vi "canDataSort.vi"() -> ()   [LabVIEW 2023] (continued)
00000004    8        68\t00\t97\tCC\t00\t16\t39\t78\r\n      1882  1FFFFFFF   00000004    8        00\t20\tFF\tFF\tFF\tFF\tFF\tFF\r\n      1872  1FFFFFFF   00000004    8        00\t20\tFF\tFF\tFF\tFF\tFF\tFF\r\n      1863  0CF102A7   00000004    8        30\t75\tE0\t2E\t80\tFF\tFF\tFD\r\n      1863  0CF101A7   00000004    8        68\t00\t97\tCC\t00\t16\t39\t77\r\n      1862  1FFFFFFF   00000004    8        00\t20\tFF\tFF\tFF\tFF\tFF\tFF\r\n      1852  1FFFFFFF   00000004    8        00\t20\tFF\tFF\tFF\tFF\tFF\tFF\r\n      1847  1FFFFFFF   00000004    8        00\t00\tFF\tFF\tFF\tFF\tFF\tFF\r\n      1846  18F121F0   00000004    8        09\t18\t00\t00\tFF\tFF\tB0\t01\r\n      1845  18F106A7   00000004    8        00\tF7\tFF\tFF\tFF\tFF\tFF\t95\r\n      1892  1FFFFFFF   00000004    8        00\t00\tFF\tFF\tFF\tFF\tFF\tFF\r\n      1883  0CF102A7   00000004    8        30\t75\tE0\t2E\t80\tFF\tFF\tFD\r\n      1883  0CF101A7   00000004    8        68\t00\t97\tCC\t00\t16\t39\t78\r\n      1882  1FFFFFFF   00000004    8        00\t20\tFF\tFF\tFF\tFF\tFF\tFF\r\n      1872  1FFFFFFF   00000004    8        00\t20\tFF\tFF\tFF\tFF\tFF\tFF\r\n      1863  0CF102A7   00000004    8        30\t75\tE0\t2E\t80\tFF\tFF\tFD\r\n      1863  0CF101A7   00000004    8        68\t00\t97\tCC\t00\t16\t39\t77\r\n      1862  1FFFFFFF   00000004    8        00\t20\tFF\tFF\tFF\tFF\tFF\tFF\r\n      1852  1FFFFFFF   00000004    8        00\t20\tFF\tFF\tFF\tFF\tFF\tFF\r\n      1847  1FFFFFFF   00000004    8        00\t00\tFF\tFF\tFF\tFF\tFF\tFF\r\n      1846  18F121F0   00000004    8        09\t18\t00\t00\tFF\tFF\tB0\t01\r\n      1893  18F106A7   00000004    8        00\tF7\tFF\tFF\tFF\tFF\tFF\t96\r\n      1892  1FFFFFFF   00000004    8        00\t00\tFF\tFF\tFF\tFF\tFF\tFF\r\n      1883  0CF102A7   00000004    8        30\t75\tE0\t2E\t80\tFF\tFF\tFD\r\n      1883  0CF101A7   00000004    8        68\t00\t97\tCC\t00\t16\t39\t78\r\n      1882  1FFFFFFF   00000004    8        00\t20\tFF\tFF\tFF\tFF\tFF\tFF\r\n      1872  1FFFFFFF   00000004    8        00\t20\tFF\tFF\tFF\tFF\tFF\tFF\r\n      1863  0CF102A7   00000004    8        30\t75\tE0\t2E\t80\tFF\tFF\tFD\r\n      1863  0CF101A7   00000004    8        68\t00\t97\tCC\t00\t16\t39\t77\r\n      1862  1FFFFFFF   00000004    8        00\t20\tFF\tFF\tFF\tFF\tFF\tFF\r\n      1852  1FFFFFFF   00000004    8        00\t20\tFF\tFF\tFF\tFF\tFF\tFF\r\n      1847  1FFFFFFF   00000004    8        00\t00\tFF\tFF\tFF\tFF\tFF\tFF\r\n      1902  1FFFFFFF   00000004    8        00\t20\tFF\tFF\tFF\tFF\tFF\tFF\r\n      1893  18F106A7   00000004    8        00\tF7\tFF\tFF\tFF\tFF\tFF\t96\r\n      1892  1FFFFFFF   00000004    8        00\t00\tFF\tFF\tFF\tFF\tFF\tFF\r\n      1883  0CF102A7   00000004    8        30\t75\tE0\t2E\t80\tFF\tFF\tFD\r\n      1883  0CF101A7   00000004    8        68\t00\t97\tCC\t00\t16\t39\t78\r\n      1882  1FFFFFFF   00000004    8        00\t20\tFF\tFF\tFF\tFF\tFF\tFF\r\n      1872  1FFFFFFF   00000004    8        00\t20\tFF\tFF\tFF\tFF\tFF\tFF\r\n      1863  0CF102A7   00000004    8        30\t75\tE0\t2E\t80\tFF\tFF\tFD\r\n      1863  0CF101A7   00000004    8        68\t00\t97\tCC\t00\t16\t39\t77\r\n      1862  1FFFFFFF   00000004    8        00\t20\tFF\tFF\tFF\tFF\tFF\tFF\r\n      1852  1FFFFFFF   00000004    8        00\t20\tFF\tFF\tFF\tFF\tFF\tFF\r\n      1903  0CF101A7   00000004    8        68\t00\t97\tCC\t00\t16\t39\t79\r\n      1902  1FFFFFFF   00000004    8        00\t20\tFF\tFF\tFF\tFF\tFF\tFF\r\n      1893  18F106A7   00000004    8        00\tF7\tFF\tFF\tFF\tFF\tFF\t96\r\n      1892  1FFFFFFF   00000004    8        00\t00\tFF\tFF\tFF\tFF\tFF\tFF\r\n      1883  0CF102A7   00000004    8        30\t75\tE0\t2E\t80\tFF\tFF\tFD\r\n      1883  0CF101A7   00000004    8        68\t00\t97\tCC\t00\t16\t39\t78\r\n      1882  1FFFFFFF   00000004    8        00\t20\tFF\tFF\tFF\tFF\tFF\tFF\r\n      1872  1FFFFFFF   00000004    8        00\t20\tFF\tFF\tFF\tFF\tFF\tFF\r\n      1863  0CF102A7   00000004    8        30\t75\tE0\t2E\t80\tFF\tFF\tFD\r\n      1863  0CF101A7   00000004    8        68\t00\t97\tCC\t00\t16\t39\t77\r\n      1862  1FFFFFFF   00000004    8        00\t20\tFF\tFF\tFF\tFF\tFF\tFF\r\n      1903  0CF102A7   00000004    8        30\t75\tE0\t2E\t80\tFF\tFF\tFD\r\n      1903  0CF101A7   00000004    8        68\t00\t97\tCC\t00\t16\t39\t79\r\n      1902  1FFFFFFF   00000004    8        00\t20\tFF\tFF\tFF\tFF\tFF\tFF\r\n      1893  18F106A7   00000004    8        00\tF7\tFF\tFF\tFF\tFF\tFF\t96\r\n      1892  1FFFFFFF   00000004    8        00\t00\tFF\tFF\tFF\tFF\tFF\tFF\r\n      1883  0CF102A7   00000004    8        30\t75\tE0\t2E\t80\tFF\tFF\tFD\r\n      1883  0CF101A7   00000004    8        68\t00\t97\tCC\t00\t16\t39\t78\r\n      1882  1FFFFFFF   00000004    8        00\t20\tFF\tFF\tFF\tFF\tFF\tFF\r\n      1872  1FFFFFFF   00000004    8        00\t20\tFF\tFF\tFF\tFF\tFF\tFF\r\n      1863  0CF102A7   00000004    8        30\t75\tE0\t2E\t80\tFF\tFF\tFD\r\n      1863  0CF101A7   00000004    8        68\t00\t97\tCC\t00\t16\t39\t77\r\n      1912  1FFFFFFF   00000004    8        00\t00\tFF\tFF\tFF\tFF\tFF\tFF\r\n      1903  0CF102A7   00000004    8        30\t75\tE0\t2E\t80\tFF\tFF\tFD\r\n      1903  0CF101A7   00000004    8        68\t00\t97\tCC\t00\t16\t39\t79\r\n      1902  1FFFFFFF   00000004    8        00\t20\tFF\tFF\tFF\tFF\tFF\tFF\r\n      1893  18F106A7   00000004    8        00\tF7\tFF\tFF\tFF\tFF\tFF\t96\r\n      1892  1FFFFFFF   00000004    8        00\t00\tFF\tFF\tFF\tFF\tFF\tFF\r\n      1883  0CF102A7   00000004    8        30\t75\tE0\t2E\t80\tFF\tFF\tFD\r\n      1883  0CF101A7   00000004    8        68\t00\t97\tCC\t00\t16\t39\t78\r\n      1882  1FFFFFFF   00000004    8        00\t20\tFF\tFF\tFF\tFF\tFF\tFF\r\n      1872  1FFFFFFF   00000004    8        00\t20\tFF\tFF\tFF\tFF\tFF\tFF\r\n      1863  0CF102A7   00000004    8        30\t75\tE0\t2E\t80\tFF\tFF\tFD\r\n      1922  1FFFFFFF   00000004    8        00\t20\tFF\tFF\tFF\tFF\tFF\tFF\r\n      1912  1FFFFFFF   00000004    8        00\t00\tFF\tFF\tFF\tFF\tFF\tFF\r\n      1903  0CF102A7   00000004    8        30\t75\tE0\t2E\t80\tFF\tFF\tFD\r\n      1903  0CF101A7   00000004    8        68\t00\t97\tCC\t00\t16\t39\t79\r\n      1902  1FFFFFFF   00000004    8        00\t20\tFF\tFF\tFF\tFF\tFF\tFF\r\n      1893  18F106A7   00000004    8        00\tF7\tFF\tFF\tFF\tFF\tFF\t96\r\n      1892  1FFFFFFF   00000004    8        00\t00\tFF\tFF\tFF\tFF\tFF\tFF\r\n      1883  0CF102A7   00000004    8        30\t75\tE0\t2E\t80\tFF\tFF\tFD\r\n      1883  0CF101A7   00000004    8        68\t00\t97\tCC\t00\t16\t39\t78\r\n      1882  1FFFFFFF   00000004    8        00\t20\tFF\tFF\tFF\tFF\tFF\tFF\r\n      1872  1FFFFFFF   00000004    8        00\t20\tFF\tFF\tFF\tFF\tFF\tFF\r\n      1923  0CF101A7   00000004    8        68\t00\t97\tCC\t00\t16\t39\t7A\r\n      1922  1FFFFFFF   00000004    8        00\t20\tFF\tFF\tFF\tFF\tFF\tFF\r\n      1912  1FFFFFFF   00000004    8        00\t00\tFF\tFF\tFF\tFF\tFF\tFF\r\n      1903  0CF102A7   00000004    8        30\t75\tE0\t2E\t80\tFF\tFF\tFD\r\n      1903  0CF101A7   00000004    8        68\t00\t97\tCC\t00\t16\t39\t79\r\n      1902  1FFFFFFF   00000004    8        00\t20\tFF\tFF\tFF\tFF\tFF\tFF\r\n      1893  18F106A7   00000004    8        00\tF7\tFF\tFF\tFF\tFF\tFF\t96\r\n      1892  1FFFFFFF   00000004    8        00\t00\tFF\tFF\tFF\tFF\tFF\tFF\r\n      1883  0CF102A7   00000004    8        30\t75\tE0\t2E\t80\tFF\tFF\tFD\r\n      1883  0CF101A7   00000004    8        68\t00\t97\tCC\t00\t16\t39\t78\r\n      1882  1FFFFFFF   00000004    8        00\t20\tFF\tFF\tFF\tFF\tFF\tFF\r\n      1923  0CF102A7   00000004    8        30\t75\tE0\t2E\t80\tFF\tFF\tFD\r\n      1923  0CF101A7   00000004    8        68\t00\t97\tCC\t00\t16\t39\t7A\r\n      1922  1FFFFFFF   00000004    8        00\t20\tFF\tFF\tFF\tFF\tFF\tFF\r\n      1912  1FFFFFFF   00000004    8        00\t00\tFF\tFF\tFF\tFF\tFF\tFF\r\n      1903  0CF102A7   00000004    8        30\t75\tE0\t2E\t80\tFF\tFF\tFD\r\n      1903  0CF101A7   00000004    8        68\t00\t97\tCC\t00\t16\t39\t79\r\n      1902  1FFFFFFF   00000004    8        00\t20\tFF\tFF\tFF\tFF\tFF\tFF\r\n      1893  18F106A7   00000004    8        00\tF7\tFF\tFF\tFF\tFF\tFF\t96\r\n      1892  1FFFFFFF   00000004    8        00\t00\tFF\tFF\tFF\tFF\tFF\tFF\r\n      1883  0CF102A7   00000004    8        30\t75\tE0\t2E\t80\tFF\tFF\tFD\r\n      1883  0CF101A7   00000004    8        68\t00\t97\tCC\t00\t16\t39\t78\r\n      1932  1FFFFFFF   00000004    8        00\t20\tFF\tFF\tFF\tFF\tFF\tFF\r\n      1923  0CF102A7   00000004    8        30\t75\tE0\t2E\t80\tFF\tFF\tFD\r\n      1923  0CF101A7   00000004    8        68\t00\t97\tCC\t00\t16\t39\t7A\r\n      1922  1FFFFFFF   00000004    8        00\t20\tFF\tFF\tFF\tFF\tFF\tFF\r\n      1912  1FFFFFFF   00000004    8        00\t00\tFF\tFF\tFF\tFF\tFF\tFF\r\n      1903  0CF102A7   00000004    8        30\t75\tE0\t2E\t80\tFF\tFF\tFD\r\n      1903  0CF101A7   00000004    8        68\t00\t97\tCC\t00\t16\t39\t79\r\n      1902  1FFFFFFF   00000004    8        00\t20\tFF\tFF\tFF\tFF\tFF\tFF\r\n      1893  18F106A7   00000004    8        00\tF7\tFF\tFF\tFF\tFF\tFF\t96\r\n      1892  1FFFFFFF   00000004    8        00\t00\tFF\tFF\tFF\tFF\tFF\tFF\r\n      1883  0CF102A7   00000004    8        30\t75\tE0\t2E\t80\tFF\tFF\tFD\r\n      1941  18F11FF0   00000004    8        FF\t3F\t90\t68\t88\t1B\t10\tBC\r\n      1932  1FFFFFFF   00000004    8        00\t20\tFF\tFF\tFF\tFF\tFF\tFF\r\n      1923  0CF102A7   00000004    8        30\t75\tE0\t2E\t80\tFF\tFF\tFD\r\n      1923  0CF101A7   00000004    8        68\t00\t97\tCC\t00\t16\t39\t7A\r\n      1922  1FFFFFFF   00000004    8        00\t20\tFF\tFF\tFF\tFF\tFF\tFF\r\n      1912  1FFFFFFF   00000004    8        00\t00\tFF\tFF\tFF\tFF\tFF\tFF\r\n      1903  0CF102A7   00000004    8        30\t75\tE0\t2E\t80\tFF\tFF\tFD\r\n      1903  0CF101A7   00000004    8        68\t00\t97\tCC\t00\t16\t39\t79\r\n      1902  1FFFFFFF   00000004    8        00\t20\tFF\tFF\tFF\tFF\tFF\tFF\r\n      1893  18F106A7   00000004    8        00\tF7\tFF\tFF\tFF\tFF\tFF\t96\r\n      1892  1FFFFFFF   00000004    8        00\t00\tFF\tFF\tFF\tFF\tFF\tFF\r\n      1942  18F120F0   00000004    8        2B\t75\t60\tB1\tB0\t01\tFF\tFF\r\n      1941  18F11FF0   00000004    8        FF\t3F\t90\t68\t88\t1B\t10\tBC\r\n      1932  1FFFFFFF   00000004    8        00\t20\tFF\tFF\tFF\tFF\tFF\tFF\r\n      1923  0CF102A7   00000004    8        30\t75\tE0\t2E\t80\tFF\tFF\tFD\r\n      1923  0CF101A7   00000004    8        68\t00\t97\tCC\t00\t16\t39\t7A\r\n      1922  1FFFFFFF   00000004    8        00\t20\tFF\tFF\tFF\tFF\tFF\tFF\r\n      1912  1FFFFFFF   00000004    8        00\t00\tFF\tFF\tFF\tFF\tFF\tFF\r\n      1903  0CF102A7   00000004    8        30\t75\tE0\t2E\t80\tFF\tFF\tFD\r\n      1903  0CF101A7   00000004    8        68\t00\t97\tCC\t00\t16\t39\t79\r\n      1902  1FFFFFFF   00000004    8        00\t20\tFF\tFF\tFF\tFF\tFF\tFF\r\n      1893  18F106A7   00000004    8        00\tF7\tFF\tFF\tFF\tFF\tFF\t96\r\n      1943  0CF101A7   00000004    8        68\t00\t97\tCC\t00\t16\t39\t7B\r\n      1942  18F120F0   00000004    8        2B\t75\t60\tB1\tB0\t01\tFF\tFF\r\n      1941  18F11FF0   00000004    8        FF\t3F\t90\t68\t88\t1B\t10\tBC\r\n      1932  1FFFFFFF   00000004    8        00\t20\tFF\tFF\tFF\tFF\tFF\tFF\r\n      1923  0CF102A7   00000004    8        30\t75\tE0\t2E\t80\tFF\tFF\tFD\r\n      1923  0CF101A7   00000004    8        68\t00\t97\tCC\t00\t16\t39\t7A\r\n      1922  1FFFFFFF   00000004    8        00\t20\tFF\tFF\tFF\tFF\tFF\tFF\r\n      1912  1FFFFFFF   00000004    8        00\t00\tFF\tFF\tFF\tFF\tFF\tFF\r\n      1903  0CF102A7   00000004    8        30\t75\tE0\t2E\t80\tFF\tFF\tFD\r\n      1903  0CF101A7   00000004    8        68\t00\t97\tCC\t00\t16\t39\t79\r\n      1902  1FFFFFFF   00000004    8        00\t20\tFF\tFF\tFF\tFF\tFF\tFF\r\n      1943  0C3C4D4A   00000004    8        BE\tFF\tFF\t7F\t18\tFF\tFF\t4B\r\n      1943  0CF101A7   00000004    8        68\t00\t97\tCC\t00\t16\t39\t7B\r\n      1942  18F120F0   00000004    8        2B\t75\t60\tB1\tB0\t01\tFF\tFF\r\n      1941  18F11FF0   00000004    8        FF\t3F\t90\t68\t88\t1B\t10\tBC\r\n      1932  1FFFFFFF   00000004    8        00\t20\tFF\tFF\tFF\tFF\tFF\tFF\r\n      1923  0CF102A7   00000004    8        30\t75\tE0\t2E\t80\tFF\tFF\tFD\r\n      1923  0CF101A7   00000004    8        68\t00\t97\tCC\t00\t16\t39\t7A\r\n      1922  1FFFFFFF   00000004    8        00\t20\tFF\tFF\tFF\tFF\tFF\tFF\r\n      1912  1FFFFFFF   00000004    8        00\t00\tFF\tFF\tFF\tFF\tFF\tFF\r\n      1903  0CF102A7   00000004    8        30\t75\tE0\t2E\t80\tFF\tFF\tFD\r\n      1903  0CF101A7   00000004    8        68\t00\t97\tCC\t00\t16\t39\t79\r\n      1944  0CF102A7   00000004    8        30\t75\tE0\t2E\t80\tFF\tFF\tFD\r\n      1943  0C3C4D4A   00000004    8        BE\tFF\tFF\t7F\t18\tFF\tFF\t4B\r\n      1943  0CF101A7   00000004    8        68\t00\t97\tCC\t00\t16\t39\t7B\r\n      1942  18F120F0   00000004    8        2B\t75\t60\tB1\tB0\t01\tFF\tFF\r\n      1941  18F11FF0   00000004    8        FF\t3F\t90\t68\t88\t1B\t10\tBC\r\n      1932  1FFFFFFF   00000004    8        00\t20\tFF\tFF\tFF\tFF\tFF\tFF\r\n      1923  0CF102A7   00000004    8        30\t75\tE0\t2E\t80\tFF\tFF\tFD\r\n      1923  0CF101A7   00000004    8        68\t00\t97\tCC\t00\t16\t39\t7A\r\n      1922  1FFFFFFF   00000004    8        00\t20\tFF\tFF\tFF\tFF\tFF\tFF\r\n      1912  1FFFFFFF   00000004    8        00\t00\tFF\tFF\tFF\tFF\tFF\tFF\r\n      1903  0CF102A7   00000004    8        30\t75\tE0\t2E\t80\tFF\tFF\tFD\r\n      1944  0CF103A7   00000004    8        17\t1F\t08\t60\tB1\t1F\t08\t4B\r\n      1944  0CF102A7   00000004    8        30\t75\tE0\t2E\t80\tFF\tFF\tFD\r\n      1943  0C3C4D4A   00000004    8        BE\tFF\tFF\t7F\t18\tFF\tFF\t4B\r\n      1943  0CF101A7   00000004    8        68\t00\t97\tCC\t00\t16\t39\t7B\r\n      1942  18F120F0   00000004    8        2B\t75\t60\tB1\tB0\t01\tFF\tFF\r\n      1941  18F11FF0   00000004    8        FF\t3F\t90\t68\t88\t1B\t10\tBC\r\n      1932  1FFFFFFF   00000004    8        00\t20\tFF\tFF\tFF\tFF\tFF\tFF\r\n      1923  0CF102A7   00000004    8        30\t75\tE0\t2E\t80\tFF\tFF\tFD\r\n      1923  0CF101A7   00000004    8        68\t00\t97\tCC\t00\t16\t39\t7A\r\n      1922  1FFFFFFF   00000004    8        00\t20\tFF\tFF\tFF\tFF\tFF\tFF\r\n      1912  1FFFFFFF   00000004    8        00\t00\tFF\tFF\tFF\tFF\tFF\tFF\r\n      1945  0CF104A7   00000004    8        F0\t60\t22\tFC\tFF\tFF\tFF\t4B\r\n      1944  0CF103A7   00000004    8        17\t1F\t08\t60\tB1\t1F\t08\t4B\r\n      1944  0CF102A7   00000004    8        30\t75\tE0\t2E\t80\tFF\tFF\tFD\r\n      1943  0C3C4D4A   00000004    8        BE\tFF\tFF\t7F\t18\tFF\tFF\t4B\r\n      1943  0CF101A7   00000004    8        68\t00\t97\tCC\t00\t16\t39\t7B\r\n      1942  18F120F0   00000004    8        2B\t75\t60\tB1\tB0\t01\tFF\tFF\r\n      1941  18F11FF0   00000004    8        FF\t3F\t90\t68\t88\t1B\t10\tBC\r\n      1932  1FFFFFFF   00000004    8        00\t20\tFF\tFF\tFF\tFF\tFF\tFF\r\n      1923  0CF102A7   00000004    8        30\t75\tE0\t2E\t80\tFF\tFF\tFD\r\n      1923  0CF101A7   00000004    8        68\t00\t97\tCC\t00\t16\t39\t7A\r\n      1922  1FFFFFFF   00000004    8        00\t20\tFF\tFF\tFF\tFF\tFF\tFF\r\n      1945  18F106A7   00000004    8        00\tF7\tFF\tFF\tFF\tFF\tFF\t97\r\n      1945  0CF104A7   00000004    8        F0\t60\t22\tFC\tFF\tFF\tFF\t4B\r\n      1944  0CF103A7   00000004    8        17\t1F\t08\t60\tB1\t1F\t08\t4B\r\n      1944  0CF102A7   00000004    8        30\t75\tE0\t2E\t80\tFF\tFF\tFD\r\n      1943  0C3C4D4A   00000004    8        BE\tFF\tFF\t7F\t18\tFF\tFF\t4B\r\n      1943  0CF101A7   00000004    8        68\t00\t97\tCC\t00\t16\t39\t7B\r\n      1942  18F120F0   00000004    8        2B\t75\t60\tB1\tB0\t01\tFF\tFF\r\n      1941  18F11FF0   00000004    8        FF\t3F\t90\t68\t88\t1B\t10\tBC\r\n      1932  1FFFFFFF   00000004    8        00\t20\tFF\tFF\tFF\tFF\tFF\tFF\r\n      1923  0CF102A7   00000004    8        30\t75\tE0\t2E\t80\tFF\tFF\tFD\r\n      1923  0CF101A7   00000004    8        68\t00\t97\tCC\t00\t16\t39\t7A\r\n      1946  18F121F0   00000004    8        09\t18\t00\t00\tFF\tFF\tB0\t01\r\n      1945  18F106A7   00000004    8        00\tF7\tFF\tFF\tFF\tFF\tFF\t97\r\n      1945  0CF104A7   00000004    8        F0\t60\t22\tFC\tFF\tFF\tFF\t4B\r\n      1944  0CF103A7   00000004    8        17\t1F\t08\t60\tB1\t1F\t08\t4B\r\n      1944  0CF102A7   00000004    8        30\t75\tE0\t2E\t80\tFF\tFF\tFD\r\n      1943  0C3C4D4A   00000004    8        BE\tFF\tFF\t7F\t18\tFF\tFF\t4B\r\n      1943  0CF101A7   00000004    8        68\t00\t97\tCC\t00\t16\t39\t7B\r\n      1942  18F120F0   00000004    8        2B\t75\t60\tB1\tB0\t01\tFF\tFF\r\n      1941  18F11FF0   00000004    8        FF\t3F\t90\t68\t88\t1B\t10\tBC\r\n      1932  1FFFFFFF   00000004    8        00\t20\tFF\tFF\tFF\tFF\tFF\tFF\r\n      1923  0CF102A7   00000004    8        30\t75\tE0\t2E\t80\tFF\tFF\tFD\r\n      1947  1FFFFFFF   00000004    8        00\t20\tFF\tFF\tFF\tFF\tFF\tFF\r\n      1946  18F121F0   00000004    8        09\t18\t00\t00\tFF\tFF\tB0\t01\r\n      1945  18F106A7   00000004    8        00\tF7\tFF\tFF\tFF\tFF\tFF\t97\r\n      1945  0CF104A7   00000004    8        F0\t60\t22\tFC\tFF\tFF\tFF\t4B\r\n      1944  0CF103A7   00000004    8        17\t1F\t08\t60\tB1\t1F\t08\t4B\r\n      1944  0CF102A7   00000004    8        30\t75\tE0\t2E\t80\tFF\tFF\tFD\r\n      1943  0C3C4D4A   00000004    8        BE\tFF\tFF\t7F\t18\tFF\tFF\t4B\r\n      1943  0CF101A7   00000004    8        68\t00\t97\tCC\t00\t16\t39\t7B\r\n      1942  18F120F0   00000004    8        2B\t75\t60\tB1\tB0\t01\tFF\tFF\r\n      1941  18F11FF0   00000004    8        FF\t3F\t90\t68\t88\t1B\t10\tBC\r\n      1932  1FFFFFFF   00000004    8        00\t20\tFF\tFF\tFF\tFF\tFF\tFF\r\n      1952  1FFFFFFF   00000004    8        00\t00\tFF\tFF\tFF\tFF\tFF\tFF\r\n      1947  1FFFFFFF   00000004    8        00\t20\tFF\tFF\tFF\tFF\tFF\tFF\r\n      1946  18F121F0   00000004    8        09\t18\t00\t00\tFF\tFF\tB0\t01\r\n      1945  18F106A7   00000004    8        00\tF7\tFF\tFF\tFF\tFF\tFF\t97\r\n      1945  0CF104A7   00000004    8        F0\t60\t22\tFC\tFF\tFF\tFF\t4B\r\n      1944  0CF103A7   00000004    8        17\t1F\t08\t60\tB1\t1F\t08\t4B\r\n      1944  0CF102A7   00000004    8        30\t75\tE0\t2E\t80\tFF\tFF\tFD\r\n      1943  0C3C4D4A   00000004    8        BE\tFF\tFF\t7F\t18\tFF\tFF\t4B\r\n      1943  0CF101A7   00000004    8        68\t00\t97\tCC\t00\t16\t39\t7B\r\n      1942  18F120F0   00000004    8        2B\t75\t60\tB1\tB0\t01\tFF\tFF\r\n      1941  18F11FF0   00000004    8        FF\t3F\t90\t68\t88\t1B\t10\tBC\r\n      1962  1FFFFFFF   00000004    8        00\t00\tFF\tFF\tFF\tFF\tFF\tFF\r\n      1952  1FFFFFFF   00000004    8        00\t00\tFF\tFF\tFF\tFF\tFF\tFF\r\n      1947  1FFFFFFF   00000004    8        00\t20\tFF\tFF\tFF\tFF\tFF\tFF\r\n      1946  18F121F0   00000004    8        09\t18\t00\t00\tFF\tFF\tB0\t01\r\n      1945  18F106A7   00000004    8        00\tF7\tFF\tFF\tFF\tFF\tFF\t97\r\n      1945  0CF104A7   00000004    8        F0\t60\t22\tFC\tFF\tFF\tFF\t4B\r\n      1944  0CF103A7   00000004    8        17\t1F\t08\t60\tB1\t1F\t08\t4B\r\n      1944  0CF102A7   00000004    8        30\t75\tE0\t2E\t80\tFF\tFF\tFD\r\n      1943  0C3C4D4A   00000004    8        BE\tFF\tFF\t7F\t18\tFF\tFF\t4B\r\n      1943  0CF101A7   00000004    8        68\t00\t97\tCC\t00\t16\t39\t7B\r\n      1942  18F120F0   00000004    8        2B\t75\t60\tB1\tB0\t01\tFF\tFF\r\n      1963  0CF101A7   00000004    8        68\t00\t97\tCC\t00\t16\t39\t7C\r\n      1962  1FFFFFFF   00000004    8        00\t00\tFF\tFF\tFF\tFF\tFF\tFF\r\n      1952  1FFFFFFF   00000004    8        00\t00\tFF\tFF\tFF\tFF\tFF\tFF\r\n      1947  1FFFFFFF   00000004    8        00\t20\tFF\tFF\tFF\tFF\tFF\tFF\r\n      1946  18F121F0   00000004    8        09\t18\t00\t00\tFF\tFF\tB0\t01\r\n      1945  18F106A7   00000004    8        00\tF7\tFF\tFF\tFF\tFF\tFF\t97\r\n      1945  0CF104A7   00000004    8        F0\t60\t22\tFC\tFF\tFF\tFF\t4B\r\n      1944  0CF103A7   00000004    8        17\t1F\t08\t60\tB1\t1F\t08\t4B\r\n      1944  0CF102A7   00000004    8        30\t75\tE0\t2E\t80\tFF\tFF\tFD\r\n      1943  0C3C4D4A   00000004    8        BE\tFF\tFF\t7F\t18\tFF\tFF\t4B\r\n      1943  0CF101A7   00000004    8        68\t00\t97\tCC\t00\t16\t39\t7B\r\n      1963  0CF102A7   00000004    8        30\t75\tE0\t2E\t80\tFF\tFF\tFD\r\n      1963  0CF101A7   00000004    8        68\t00\t97\tCC\t00\t16\t39\t7C\r\n      1962  1FFFFFFF   00000004    8        00\t00\tFF\tFF\tFF\tFF\tFF\tFF\r\n      1952  1FFFFFFF   00000004    8        00\t00\tFF\tFF\tFF\tFF\tFF\tFF\r\n      1947  1FFFFFFF   00000004    8        00\t20\tFF\tFF\tFF\tFF\tFF\tFF\r\n      1946  18F121F0   00000004    8        09\t18\t00\t00\tFF\tFF\tB0\t01\r\n      1945  18F106A7   00000004    8        00\tF7\tFF\tFF\tFF\tFF\tFF\t97\r\n      1945  0CF104A7   00000004    8        F0\t60\t22\tFC\tFF\tFF\tFF\t4B\r\n      1944  0CF103A7   00000004    8        17\t1F\t08\t60\tB1\t1F\t08\t4B\r\n      1944  0CF102A7   00000004    8        30\t75\tE0\t2E\t80\tFF\tFF\tFD\r\n      1943  0C3C4D4A   00000004    8        BE\tFF\tFF\t7F\t18\tFF\tFF\t4B\r\n      1972  1FFFFFFF   00000004    8        00\t00\tFF\tFF\tFF\tFF\tFF\tFF\r\n      1963  0CF102A7   00000004    8        30\t75\tE0\t2E\t80\tFF\tFF\tFD\r\n      1963  0CF101A7   00000004    8        68\t00\t97\tCC\t00\t16\t39\t7C\r\n      1962  1FFFFFFF   00000004    8        00\t00\tFF\tFF\tFF\tFF\tFF\tFF\r\n      1952  1FFFFFFF   00000004    8        00\t00\tFF\tFF\tFF\tFF\tFF\tFF\r\n      1947  1FFFFFFF   00000004    8        00\t20\tFF\tFF\tFF\tFF\tFF\tFF\r\n      1946  18F121F0   00000004    8        09\t18\t00\t00\tFF\tFF\tB0\t01\r\n      1945  18F106A7   00000004    8        00\tF7\tFF\tFF\tFF\tFF\tFF\t97\r\n      1945  0CF104A7   00000004    8        F0\t60\t22\tFC\tFF\tFF\tFF\t4B\r\n      1944  0CF103A7   00000004    8        17\t1F\t08\t60\tB1\t1F\t08\t4B\r\n      1944  0CF102A7   00000004    8        30\t75\tE0\t2E\t80\tFF\tFF\tFD\r\n      1982  1FFFFFFF   00000004    8        00\t20\tFF\tFF\tFF\tFF\tFF\tFF\r\n      1972  1FFFFFFF   00000004    8        00\t00\tFF\tFF\tFF\tFF\tFF\tFF\r\n      1963  0CF102A7   00000004    8        30\t75\tE0\t2E\t80\tFF\tFF\tFD\r\n      1963  0CF101A7   00000004    8        68\t00\t97\tCC\t00\t16\t39\t7C\r\n      1962  1FFFFFFF   00000004    8        00\t00\tFF\tFF\tFF\tFF\tFF\tFF\r\n      1952  1FFFFFFF   00000004    8        00\t00\tFF\tFF\tFF\tFF\tFF\tFF\r\n      1947  1FFFFFFF   00000004    8        00\t20\tFF\tFF\tFF\tFF\tFF\tFF\r\n      1946  18F121F0   00000004    8        09\t18\t00\t00\tFF\tFF\tB0\t01\r\n      1945  18F106A7   00000004    8        00\tF7\tFF\tFF\tFF\tFF\tFF\t97\r\n      1945  0CF104A7   00000004    8        F0\t60\t22\tFC\tFF\tFF\tFF\t4B\r\n      1944  0CF103A7   00000004    8        17\t1F\t08\t60\tB1\t1F\t08\t4B\r\n      1983  0CF101A7   00000004    8        68\t00\t97\tCC\t00\t16\t39\t7D\r\n      1982  1FFFFFFF   00000004    8        00\t20\tFF\tFF\tFF\tFF\tFF\tFF\r\n      1972  1FFFFFFF   00000004    8        00\t00\tFF\tFF\tFF\tFF\tFF\tFF\r\n      1963  0CF102A7   00000004    8        30\t75\tE0\t2E\t80\tFF\tFF\tFD\r\n      1963  0CF101A7   00000004    8        68\t00\t97\tCC\t00\t16\t39\t7C\r\n      1962  1FFFFFFF   00000004    8        00\t00\tFF\tFF\tFF\tFF\tFF\tFF\r\n      1952  1FFFFFFF   00000004    8        00\t00\tFF\tFF\tFF\tFF\tFF\tFF\r\n      1947  1FFFFFFF   00000004    8        00\t20\tFF\tFF\tFF\tFF\tFF\tFF\r\n      1946  18F121F0   00000004    8        09\t18\t00\t00\tFF\tFF\tB0\t01\r\n      1945  18F106A7   00000004    8        00\tF7\tFF\tFF\tFF\tFF\tFF\t97\r\n      1945  0CF104A7   00000004    8        F0\t60\t22\tFC\tFF\tFF\tFF\t4B\r\n      1983  0CF102A7   00000004    8        30\t75\tE0\t2E\t80\tFF\tFF\tFD\r\n      1983  0CF101A7   00000004    8        68\t00\t97\tCC\t00\t16\t39\t7D\r\n      1982  1FFFFFFF   00000004    8        00\t20\tFF\tFF\tFF\tFF\tFF\tFF\r\n      1972  1FFFFFFF   00000004    8        00\t00\tFF\tFF\tFF\tFF\tFF\tFF\r\n      1963  0CF102A7   00000004    8        30\t75\tE0\t2E\t80\tFF\tFF\tFD\r\n      1963  0CF101A7   00000004    8        68\t00\t97\tCC\t00\t16\t39\t7C\r\n      1962  1FFFFFFF   00000004    8        00\t00\tFF\tFF\tFF\tFF\tFF\tFF\r\n      1952  1FFFFFFF   00000004    8        00\t00\tFF\tFF\tFF\tFF\tFF\tFF\r\n      1947  1FFFFFFF   00000004    8        00\t20\tFF\tFF\tFF\tFF\tFF\tFF\r\n      1946  18F121F0   00000004    8        09\t18\t00\t00\tFF\tFF\tB0\t01\r\n      1945  18F106A7   00000004    8        00\tF7\tFF\tFF\tFF\tFF\tFF\t97\r\n      1992  1FFFFFFF   00000004    8        00\t00\tFF\tFF\tFF\tFF\tFF\tFF\r\n      1983  0CF102A7   00000004    8        30\t75\tE0\t2E\t80\tFF\tFF\tFD\r\n      1983  0CF101A7   00000004    8        68\t00\t97\tCC\t00\t16\t39\t7D\r\n      1982  1FFFFFFF   00000004    8        00\t20\tFF\tFF\tFF\tFF\tFF\tFF\r\n      1972  1FFFFFFF   00000004    8        00\t00\tFF\tFF\tFF\tFF\tFF\tFF\r\n      1963  0CF102A7   00000004    8        30\t75\tE0\t2E\t80\tFF\tFF\tFD\r\n      1963  0CF101A7   00000004    8        68\t00\t97\tCC\t00\t16\t39\t7C\r\n      1962  1FFFFFFF   00000004    8        00\t00\tFF\tFF\tFF\tFF\tFF\tFF\r\n      1952  1FFFFFFF   00000004    8        00\t00\tFF\tFF\tFF\tFF\tFF\tFF\r\n      1947  1FFFFFFF   00000004    8        00\t20\tFF\tFF\tFF\tFF\tFF\tFF\r\n      1946  18F121F0   00000004    8        09\t18\t00\t00\tFF\tFF\tB0\t01\r\n      1993  18F106A7   00000004    8        00\tF7\tFF\tFF\tFF\tFF\tFF\t98\r\n      1992  1FFFFFFF   00000004    8        00\t00\tFF\tFF\tFF\tFF\tFF\tFF\r\n      1983  0CF102A7   00000004    8        30\t75\tE0\t2E\t80\tFF\tFF\tFD\r\n      1983  0CF101A7   00000004    8        68\t00\t97\tCC\t00\t16\t39\t7D\r\n      1982  1FFFFFFF   00000004    8        00\t20\tFF\tFF\tFF\tFF\tFF\tFF\r\n      1972  1FFFFFFF   00000004    8        00\t00\tFF\tFF\tFF\tFF\tFF\tFF\r\n      1963  0CF102A7   00000004    8        30\t75\tE0\t2E\t80\tFF\tFF\tFD\r\n      1963  0CF101A7   00000004    8        68\t00\t97\tCC\t00\t16\t39\t7C\r\n      1962  1FFFFFFF   00000004    8        00\t00\tFF\tFF\tFF\tFF\tFF\tFF\r\n      1952  1FFFFFFF   00000004    8        00\t00\tFF\tFF\tFF\tFF\tFF\tFF\r\n      1947  1FFFFFFF   00000004    8        00\t20\tFF\tFF\tFF\tFF\tFF\tFF\r\n      2002  1FFFFFFF   00000004    8        00\t00\tFF\tFF\tFF\tFF\tFF\tFF\r\n      1993  18F106A7   00000004    8        00\tF7\tFF\tFF\tFF\tFF\tFF\t98\r\n      1992  1FFFFFFF   00000004    8        00\t00\tFF\tFF\tFF\tFF\tFF\tFF\r\n      1983  0CF102A7   00000004    8        30\t75\tE0\t2E\t80\tFF\tFF\tFD\r\n      1983  0CF101A7   00000004    8        68\t00\t97\tCC\t00\t16\t39\t7D\r\n      1982  1FFFFFFF   00000004    8        00\t20\tFF\tFF\tFF\tFF\tFF\tFF\r\n      1972  1FFFFFFF   00000004    8        00\t00\tFF\tFF\tFF\tFF\tFF\tFF\r\n      1963  0CF102A7   00000004    8        30\t75\tE0\t2E\t80\tFF\tFF\tFD\r\n      1963  0CF101A7   00000004    8        68\t00\t97\tCC\t00\t16\t39\t7C\r\n      1962  1FFFFFFF   00000004    8        00\t00\tFF\tFF\tFF\tFF\tFF\tFF\r\n      1952  1FFFFFFF   00000004    8        00\t00\tFF\tFF\tFF\tFF\tFF\tFF\r\n      2003  0CF101A7   00000004    8        68\t00\t97\tCC\t00\t16\t39\t7E\r\n      2002  1FFFFFFF   00000004    8        00\t00\tFF\tFF\tFF\tFF\tFF\tFF\r\n      1993  18F106A7   00000004    8        00\tF7\tFF\tFF\tFF\tFF\tFF\t98\r\n      1992  1FFFFFFF   00000004    8        00\t00\tFF\tFF\tFF\tFF\tFF\tFF\r\n      1983  0CF102A7   00000004    8        30\t75\tE0\t2E\t80\tFF\tFF\tFD\r\n      1983  0CF101A7   00000004    8        68\t00\t97\tCC\t00\t16\t39\t7D\r\n      1982  1FFFFFFF   00000004    8        00\t20\tFF\tFF\tFF\tFF\tFF\tFF\r\n      1972  1FFFFFFF   00000004    8        00\t00\tFF\tFF\tFF\tFF\tFF\tFF\r\n      1963  0CF102A7   00000004    8        30\t75\tE0\t2E\t80\tFF\tFF\tFD\r\n      1963  0CF101A7   00000004    8        68\t00\t97\tCC\t00\t16\t39\t7C\r\n      1962  1FFFFFFF   00000004    8        00\t00\tFF\tFF\tFF\tFF\tFF\tFF\r\n      2003  0CF102A7   00000004    8        30\t75\tE0\t2E\t80\tFF\tFF\tFD\r\n      2003  0CF101A7   00000004    8        68\t00\t97\tCC\t00\t16\t39\t7E\r\n      2002  1FFFFFFF   00000004    8        00\t00\tFF\tFF\tFF\tFF\tFF\tFF\r\n      1993  18F106A7   00000004    8        00\tF7\tFF\tFF\tFF\tFF\tFF\t98\r\n      1992  1FFFFFFF   00000004    8        00\t00\tFF\tFF\tFF\tFF\tFF\tFF\r\n      1983  0CF102A7   00000004    8        30\t75\tE0\t2E\t80\tFF\tFF\tFD\r\n      1983  0CF101A7   00000004    8        68\t00\t97\tCC\t00\t16\t39\t7D\r\n      1982  1FFFFFFF   00000004    8        00\t20\tFF\tFF\tFF\tFF\tFF\tFF\r\n      1972  1FFFFFFF   00000004    8        00\t00\tFF\tFF\tFF\tFF\tFF\tFF\r\n      1963  0CF102A7   00000004    8        30\t75\tE0\t2E\t80\tFF\tFF\tFD\r\n      1963  0CF101A7   00000004    8        68\t00\t97\tCC\t00\t16\t39\t7C\r\n      2012  1FFFFFFF   00000004    8        00\t00\tFF\tFF\tFF\tFF\tFF\tFF\r\n      2003  0CF102A7   00000004    8        30\t75\tE0\t2E\t80\tFF\tFF\tFD\r\n      2003  0CF101A7   00000004    8        68\t00\t97\tCC\t00\t16\t39\t7E\r\n      2002  1FFFFFFF   00000004    8        00\t00\tFF\tFF\tFF\tFF\tFF\tFF\r\n      1993  18F106A7   00000004    8        00\tF7\tFF\tFF\tFF\tFF\tFF\t98\r\n      1992  1FFFFFFF   00000004    8        00\t00\tFF\tFF\tFF\tFF\tFF\tFF\r\n      1983  0CF102A7   00000004    8        30\t75\tE0\t2E\t80\tFF\tFF\tFD\r\n      1983  0CF101A7   00000004    8        68\t00\t97\tCC\t00\t16\t39\t7D\r\n      1982  1FFFFFFF   00000004    8        00\t20\tFF\tFF\tFF\tFF\tFF\tFF\r\n      1972  1FFFFFFF   00000004    8        00\t00\tFF\tFF\tFF\tFF\tFF\tFF\r\n      1963  0CF102A7   00000004    8        30\t75\tE0\t2E\t80\tFF\tFF\tFD\r\n      2022  1FFFFFFF   00000004    8        00\t00\tFF\tFF\tFF\tFF\tFF\tFF\r\n      2012  1FFFFFFF   00000004    8        00\t00\tFF\tFF\tFF\tFF\tFF\tFF\r\n      2003  0CF102A7   00000004    8        30\t75\tE0\t2E\t80\tFF\tFF\tFD\r\n      2003  0CF101A7   00000004    8        68\t00\t97\tCC\t00\t16\t39\t7E\r\n      2002  1FFFFFFF   00000004    8        00\t00\tFF\tFF\tFF\tFF\tFF\tFF\r\n      1993  18F106A7   00000004    8        00\tF7\tFF\tFF\tFF\tFF\tFF\t98\r\n      1992  1FFFFFFF   00000004    8        00\t00\tFF\tFF\tFF\tFF\tFF\tFF\r\n      1983  0CF102A7   00000004    8        30\t75\tE0\t2E\t80\tFF\tFF\tFD\r\n      1983  0CF101A7   00000004    8        68\t00\t97\tCC\t00\t16\t39\t7D\r\n      1982  1FFFFFFF   00000004    8        00\t20\tFF\tFF\tFF\tFF\tFF\tFF\r\n      1972  1FFFFFFF   00000004    8        00\t00\tFF\tFF\tFF\tFF\tFF\tFF\r\n      2023  0CF101A7   00000004    8        68\t00\t97\tCC\t00\t16\t39\t7F\r\n      2022  1FFFFFFF   00000004    8        00\t00\tFF\tFF\tFF\tFF\tFF\tFF\r\n      2012  1FFFFFFF   00000004    8        00\t00\tFF\tFF\tFF\tFF\tFF\tFF\r\n      2003  0CF102A7   00000004    8        30\t75\tE0\t2E\t80\tFF\tFF\tFD\r\n      2003  0CF101A7   00000004    8        68\t00\t97\tCC\t00\t16\t39\t7E\r\n      2002  1FFFFFFF   00000004    8        00\t00\tFF\tFF\tFF\tFF\tFF\tFF\r\n      1993  18F106A7   00000004    8        00\tF7\tFF\tFF\tFF\tFF\tFF\t98\r\n      1992  1FFFFFFF   00000004    8        00\t00\tFF\tFF\tFF\tFF\tFF\tFF\r\n      1983  0CF102A7   00000004    8        30\t75\tE0\t2E\t80\tFF\tFF\tFD\r\n      1983  0CF101A7   00000004    8        68\t00\t97\tCC\t00\t16\t39\t7D\r\n      1982  1FFFFFFF   00000004    8        00\t20\tFF\tFF\tFF\tFF\tFF\tFF\r\n      2023  0CF102A7   00000004    8        30\t75\tE0\t2E\t80\tFF\tFF\tFD\r\n      2023  0CF101A7   00000004    8        68\t00\t97\tCC\t00\t16\t39\t7F\r\n      2022  1FFFFFFF   00000004    8        00\t00\tFF\tFF\tFF\tFF\tFF\tFF\r\n      2012  1FFFFFFF   00000004    8        00\t00\tFF\tFF\tFF\tFF\tFF\tFF\r\n      2003  0CF102A7   00000004    8        30\t75\tE0\t2E\t80\tFF\tFF\tFD\r\n      2003  0CF101A7   00000004    8        68\t00\t97\tCC\t00\t16\t39\t7E\r\n      2002  1FFFFFFF   00000004    8        00\t00\tFF\tFF\tFF\tFF\tFF\tFF\r\n      1993  18F106A7   00000004    8        00\tF7\tFF\tFF\tFF\tFF\tFF\t98\r\n      1992  1FFFFFFF   00000004    8        00\t00\tFF\tFF\tFF\tFF\tFF\tFF\r\n      1983  0CF102A7   00000004    8        30\t75\tE0\t2E\t80\tFF\tFF\tFD\r\n      1983  0CF101A7   00000004    8        68\t00\t97\tCC\t00\t16\t39\t7D\r\n      2032  1FFFFFFF   00000004    8        00\t00\tFF\tFF\tFF\tFF\tFF\tFF\r\n      2023  0CF102A7   00000004    8        30\t75\tE0\t2E\t80\tFF\tFF\tFD\r\n      2023  0CF101A7   00000004    8        68\t00\t97\tCC\t00\t16\t39\t7F\r\n      2022  1FFFFFFF   00000004    8        00\t00\tFF\tFF\tFF\tFF\tFF\tFF\r\n      2012  1FFFFFFF   00000004    8        00\t00\tFF\tFF\tFF\tFF\tFF\tFF\r\n      2003  0CF102A7   00000004    8        30\t75\tE0\t2E\t80\tFF\tFF\tFD\r\n      2003  0CF101A7   00000004    8        68\t00\t97\tCC\t00\t16\t39\t7E\r\n      2002  1FFFFFFF   00000004    8        00\t00\tFF\tFF\tFF\tFF\tFF\tFF\r\n      1993  18F106A7   00000004    8        00\tF7\tFF\tFF\tFF\tFF\tFF\t98\r\n      1992  1FFFFFFF   00000004    8        00\t00\tFF\tFF\tFF\tFF\tFF\tFF\r\n      1983  0CF102A7   00000004    8        30\t75\tE0\t2E\t80\tFF\tFF\tFD\r\n      2041  18F11FF0   00000004    8        FF\t3F\t90\t68\t88\t1B\t10\tCC\r\n      2032  1FFFFFFF   00000004    8        00\t00\tFF\tFF\tFF\tFF\tFF\tFF\r\n      2023  0CF102A7   00000004    8        30\t75\tE0\t2E\t80\tFF\tFF\tFD\r\n      2023  0CF101A7   00000004    8        68\t00\t97\tCC\t00\t16\t39\t7F\r\n      2022  1FFFFFFF   00000004    8        00\t00\tFF\tFF\tFF\tFF\tFF\tFF\r\n      2012  1FFFFFFF   00000004    8        00\t00\tFF\tFF\tFF\tFF\tFF\tFF\r\n      2003  0CF102A7   00000004    8        30\t75\tE0\t2E\t80\tFF\tFF\tFD\r\n      2003  0CF101A7   00000004    8        68\t00\t97\tCC\t00\t16\t39\t7E\r\n      2002  1FFFFFFF   00000004    8        00\t00\tFF\tFF\tFF\tFF\tFF\tFF\r\n      1993  18F106A7   00000004    8        00\tF7\tFF\tFF\tFF\tFF\tFF\t98\r\n      1992  1FFFFFFF   00000004    8        00\t00\tFF\tFF\tFF\tFF\tFF\tFF\r\n      2042  18F120F0   00000004    8        2B\t75\t60\tB1\tB0\t01\tFF\tFF\r\n      2041  18F11FF0   00000004    8        FF\t3F\t90\t68\t88\t1B\t10\tCC\r\n      2032  1FFFFFFF   00000004    8        00\t00\tFF\tFF\tFF\tFF\tFF\tFF\r\n      2023  0CF102A7   00000004    8        30\t75\tE0\t2E\t80\tFF\tFF\tFD\r\n      2023  0CF101A7   00000004    8        68\t00\t97\tCC\t00\t16\t39\t7F\r\n      2022  1FFFFFFF   00000004    8        00\t00\tFF\tFF\tFF\tFF\tFF\tFF\r\n      2012  1FFFFFFF   00000004    8        00\t00\tFF\tFF\tFF\tFF\tFF\tFF\r\n      2003  0CF102A7   00000004    8        30\t75\tE0\t2E\t80\tFF\tFF\tFD\r\n      2003  0CF101A7   00000004    8        68\t00\t97\tCC\t00\t16\t39\t7E\r\n      2002  1FFFFFFF   00000004    8        00\t00\tFF\tFF\tFF\tFF\tFF\tFF\r\n      1993  18F106A7   00000004    8        00\tF7\tFF\tFF\tFF\tFF\tFF\t98\r\n      2043  0CF101A7   00000004    8        68\t00\t97\tCC\t00\t16\t39\t80\r\n      2042  18F120F0   00000004    8        2B\t75\t60\tB1\tB0\t01\tFF\tFF\r\n      2041  18F11FF0   00000004    8        FF\t3F\t90\t68\t88\t1B\t10\tCC\r\n      2032  1FFFFFFF   00000004    8        00\t00\tFF\tFF\tFF\tFF\tFF\tFF\r\n      2023  0CF102A7   00000004    8        30\t75\tE0\t2E\t80\tFF\tFF\tFD\r\n      2023  0CF101A7   00000004    8        68\t00\t97\tCC\t00\t16\t39\t7F\r\n      2022  1FFFFFFF   00000004    8        00\t00\tFF\tFF\tFF\tFF\tFF\tFF\r\n      2012  1FFFFFFF   00000004    8        00\t00\tFF\tFF\tFF\tFF\tFF\tFF\r\n      2003  0CF102A7   00000004    8        30\t75\tE0\t2E\t80\tFF\tFF\tFD\r\n      2003  0CF101A7   00000004    8        68\t00\t97\tCC\t00\t16\t39\t7E\r\n      2002  1FFFFFFF   00000004    8        00\t00\tFF\tFF\tFF\tFF\tFF\tFF\r\n      2043  0C3C4D4A   00000004    8        BE\tFF\tFF\t7F\t18\tFF\tFF\t4C\r\n      2043  0CF101A7   00000004    8        68\t00\t97\tCC\t00\t16\t39\t80\r\n      2042  18F120F0   00000004    8        2B\t75\t60\tB1\tB0\t01\tFF\tFF\r\n      2041  18F11FF0   00000004    8        FF\t3F\t90\t68\t88\t1B\t10\tCC\r\n      2032  1FFFFFFF   00000004    8        00\t00\tFF\tFF\tFF\tFF\tFF\tFF\r\n      2023  0CF102A7   00000004    8        30\t75\tE0\t2E\t80\tFF\tFF\tFD\r\n      2023  0CF101A7   00000004    8        68\t00\t97\tCC\t00\t16\t39\t7F\r\n      2022  1FFFFFFF   00000004    8        00\t00\tFF\tFF\tFF\tFF\tFF\tFF\r\n      2012  1FFFFFFF   00000004    8        00\t00\tFF\tFF\tFF\tFF\tFF\tFF\r\n      2003  0CF102A7   00000004    8        30\t75\tE0\t2E\t80\tFF\tFF\tFD\r\n      2003  0CF101A7   00000004    8        68\t00\t97\tCC\t00\t16\t39\t7E\r\n      2044  0CF102A7   00000004    8        30\t75\tE0\t2E\t80\tFF\tFF\tFD\r\n      2043  0C3C4D4A   00000004    8        BE\tFF\tFF\t7F\t18\tFF\tFF\t4C\r\n      2043  0CF101A7   00000004    8        68\t00\t97\tCC\t00\t16\t39\t80\r\n      2042  18F120F0   00000004    8        2B\t75\t60\tB1\tB0\t01\tFF\tFF\r\n      2041  18F11FF0   00000004    8        FF\t3F\t90\t68\t88\t1B\t10\tCC\r\n      2032  1FFFFFFF   00000004    8        00\t00\tFF\tFF\tFF\tFF\tFF\tFF\r\n      2023  0CF102A7   00000004    8        30\t75\tE0\t2E\t80\tFF\tFF\tFD\r\n      2023  0CF101A7   00000004    8        68\t00\t97\tCC\t00\t16\t39\t7F\r\n      2022  1FFFFFFF   00000004    8        00\t00\tFF\tFF\tFF\tFF\tFF\tFF\r\n      2012  1FFFFFFF   00000004    8        00\t00\tFF\tFF\tFF\tFF\tFF\tFF\r\n      2003  0CF102A7   00000004    8        30\t75\tE0\t2E\t80\tFF\tFF\tFD\r\n      2044  0CF103A7   00000004    8        17\t1F\t08\t60\tB1\t1F\t08\t4C\r\n      2044  0CF102A7   00000004    8        30\t75\tE0\t2E\t80\tFF\tFF\tFD\r\n      2043  0C3C4D4A   00000004    8        BE\tFF\tFF\t7F\t18\tFF\tFF\t4C\r\n      2043  0CF101A7   00000004    8        68\t00\t97\tCC\t00\t16\t39\t80\r\n      2042  18F120F0   00000004    8        2B\t75\t60\tB1\tB0\t01\tFF\tFF\r\n      2041  18F11FF0   00000004    8        FF\t3F\t90\t68\t88\t1B\t10\tCC\r\n      2032  1FFFFFFF   00000004    8        00\t00\tFF\tFF\tFF\tFF\tFF\tFF\r\n      2023  0CF102A7   00000004    8        30\t75\tE0\t2E\t80\tFF\tFF\tFD\r\n      2023  0CF101A7   00000004    8        68\t00\t97\tCC\t00\t16\t39\t7F\r\n      2022  1FFFFFFF   00000004    8        00\t00\tFF\tFF\tFF\tFF\tFF\tFF\r\n      2012  1FFFFFFF   00000004    8        00\t00\tFF\tFF\tFF\tFF\tFF\tFF\r\n      2045  0CF104A7   00000004    8        F0\t60\t22\tFC\tFF\tFF\tFF\t4C\r\n      2044  0CF103A7   00000004    8        17\t1F\t08\t60\tB1\t1F\t08\t4C\r\n      2044  0CF102A7   00000004    8        30\t75\tE0\t2E\t80\tFF\tFF\tFD\r\n      2043  0C3C4D4A   00000004    8        BE\tFF\tFF\t7F\t18\tFF\tFF\t4C\r\n      2043  0CF101A7   00000004    8        68\t00\t97\tCC\t00\t16\t39\t80\r\n      2042  18F120F0   00000004    8        2B\t75\t60\tB1\tB0\t01\tFF\tFF\r\n      2041  18F11FF0   00000004    8        FF\t3F\t90\t68\t88\t1B\t10\tCC\r\n      2032  1FFFFFFF   00000004    8        00\t00\tFF\tFF\tFF\tFF\tFF\tFF\r\n      2023  0CF102A7   00000004    8        30\t75\tE0\t2E\t80\tFF\tFF\tFD\r\n      2023  0CF101A7   00000004    8        68\t00\t97\tCC\t00\t16\t39\t7F\r\n      2022  1FFFFFFF   00000004    8        00\t00\tFF\tFF\tFF\tFF\tFF\tFF\r\n      2045  18F106A7   00000004    8        00\tF7\tFF\tFF\tFF\tFF\tFF\t99\r\n      2045  0CF104A7   00000004    8        F0\t60\t22\tFC\tFF\tFF\tFF\t4C\r\n      2044  0CF103A7   00000004    8        17\t1F\t08\t60\tB1\t1F\t08\t4C\r\n      2044  0CF102A7   00000004    8        30\t75\tE0\t2E\t80\tFF\tFF\tFD\r\n      2043  0C3C4D4A   00000004    8        BE\tFF\tFF\t7F\t18\tFF\tFF\t4C\r\n      2043  0CF101A7   00000004    8        68\t00\t97\tCC\t00\t16\t39\t80\r\n      2042  18F120F0   00000004    8        2B\t75\t60\tB1\tB0\t01\tFF\tFF\r\n      2041  18F11FF0   00000004    8        FF\t3F\t90\t68\t88\t1B\t10\tCC\r\n
